vi "Test AC Gain.vi"(8 "error in (no error)":errorcluster, 11 "SR7270 Drivers in":refnum<class "SR7270 Drivers.lvclass">) -> (0 "error out":errorcluster, 3 "SR7270 Drivers out":refnum<class "SR7270 Drivers.lvclass">)   [LabVIEW 2016, in "SR7270 Drivers.lvlib"]
uses:
  SR7270 Drivers.lvlib
  <vilib>/addons/_JKI Toolkits/Caraya/classes/Assert/Assert.lvclass
  Typedefs/SEN-IMODE0--enum.ctl
  <vilib>/addons/_JKI Toolkits/Caraya/classes/Test/Test.lvclass
  Typedefs/ACGAIN--enum.ctl
  SR7270 Drivers.lvclass
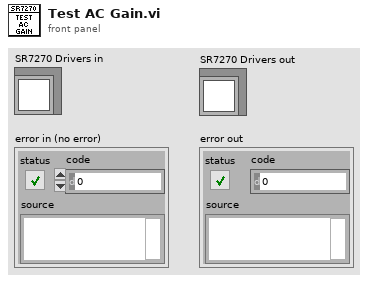
[diagram p1: front panel]
types:
  T1 = typedef "SR7270 Drivers.lvlib/ACGAIN--enum.ctl" = enum16{"0 dB", "6 dB", "12 dB", "18 dB", "24 dB", "30 dB", "36 dB", "42 dB", "48 dB", "54 dB", "60 dB", "66 dB", "72 dB", "78 dB", "84 dB", "90 dB"}
  T2 = typedef "SR7270 Drivers.lvlib/SEN-IMODE0--enum.ctl" = enum16{"2 nV", "5 nV", "10 nV", "20 nV", "50 nV", "100 nV", "200 nV", "500 nV", "1 µV", "2 µV", "5 µV", "10 µV", "20 µV", "50 µV", "100 µV", "200 µV", "500 µV", "1 mV", "2 mV", "5 mV", "10 mV", "20 mV", "50 mV", "100 mV", "200 mV", "500 mV", "1 V"}
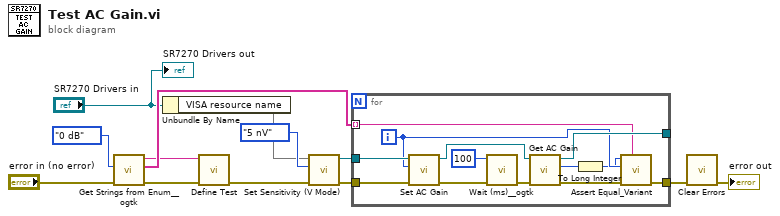
[diagram p0: block diagram]
diagram:
  n1 = call <userlib>:"Get Strings from Enum__ogtk.vi"("error in (no error)"="error in (no error)", "Enum"=ACGAIN--enum."0 dB" ("AC Gain")) -> ("error out"=w6:errorcluster, "Enum Strings"=w9:string[], "Enum Name"=w7:string)  [unwired: 6 in, 1 out]
  n2 = Unbundle By Name("SR7270 Drivers in") -> ("VISA resource name"=w2)
  n3 = call <vilib>:"Define Test.vi"("error in (no error)"=w6, "Label (VI Title)"=w7) -> ("error out"=w4:errorcluster)  [unwired: 9 in]
  n4 = call "Set Sensitivity (V Mode).vi"("error in (no error)"=w4, "Sensitivity IMODE0"=SEN-IMODE0--enum."5 nV", "VISA resource name"=w2) -> ("error out"=w3:errorcluster, "VISA resource name out"=w12:refnum<visa-resource-name>)  [unwired: 7 in]
  n5 = for {
    tunnel: w12 -> [w25]
    tunnel: w3 -> [w17]
    tunnel: [w23] -> w11
    tunnel: [w22] -> _
    tunnel: w9 -> [w14] mode=indexing
    i -> [w16]
    n6 = call "Set AC Gain.vi"("error in (no error)"=w17, "AC Gain"=w16, "VISA resource name"=w25) -> ("error out"=w19:errorcluster, "VISA resource name out"=w26:refnum<visa-resource-name>)  [unwired: 7 in]
    n7 = call <userlib>:"Wait (ms)__ogtk.vi"("error in (no error)"=w19, "milliseconds to wait"=u32 100) -> ("error out"=w21:errorcluster)  [unwired: 8 in, 1 out]
    n8 = call "Get AC Gain.vi"("error in (no error)"=w21, "VISA resource name"=w26) -> ("error out"=w24:errorcluster, "AC Gain"=w18:T1, "VISA resource name out"=w22:refnum<visa-resource-name>)  [unwired: 7 in]
    n9 = To Long Integer(number=w18) -> (32bit integer=w15:i32)
    n10 = call <vilib>:"Assert Equal_Variant.vi"("Label"=w14, "error in (no error)"=w24, "Y"=w16, "X"=w15) -> ("error out"=w23:errorcluster)  [unwired: 7 in]
  }
  n11 = call <vilib>:"Clear Errors.vi"("error in (no error)"=w11) -> ("error out"=→"error out":errorcluster)  [unwired: 5 in, 1 out]
  "SR7270 Drivers out" <- "SR7270 Drivers in"
